vi "ElevEnc.vi"(11 "Reset?":bool) -> (3 "ElevEnc":dbl)   [LabVIEW 2017]
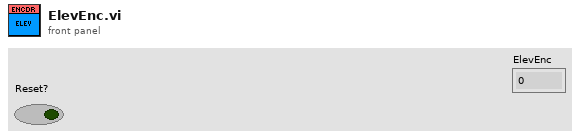
[diagram p1: front panel]
types:
  T1 = typedef "WPI_EncoderDevRef.ctl" = cluster{"DevStatus":errorcluster, "EncoderIndex":T2, "CounterIndex":T3, "DistancePerCount":dbl, "Decoding Type":T4}
  T2 = typedef "FPGA_EncoderIdx.ctl" = enum8{"Enc 0", "Enc 1", "Enc 2", "Enc 3", "Enc 4", "Enc 5", "Enc 6", "Enc 7", "Invalid"}
  T3 = typedef "FPGA_CounterCtrSystemIndex.ctl" = enum8{"Ctr 0", "Ctr 1", "Ctr 2", "Ctr 3", "Ctr 4", "Ctr 5", "Ctr 6", "Ctr 7", "Invalid"}
  T4 = typedef "WPI_EncoderType.ctl" = enum16{"1x", "2x", "4x"}
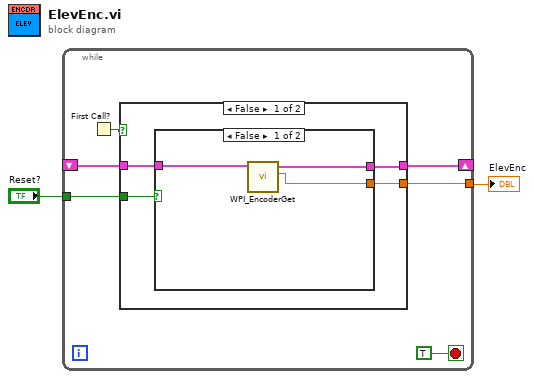
[diagram p0: block diagram]
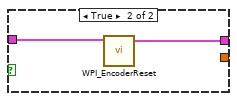
[diagram p2: hidden frame]
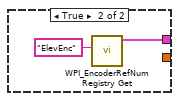
[diagram p3: hidden frame]
diagram:
  n1 = while {
    shift-right: [w6] -> _
    shift-left: _ -> [w5]
    tunnel: "Reset?" -> [w4]
    tunnel: [w3] -> w1
    stop <- TRUE stop-if-true
    n2 = First Call?() -> (First Call?: T/F=w8:bool)
    n3 = case shown="False" w8 {
      tunnel: [w10 w18] -> w6
      tunnel: w5 -> [w11 _]
      tunnel: w4 -> [w12 _]
      tunnel: [w9 _] -> w3
      frame False {
        n4 = case shown="False" w12 {
          tunnel: w11 -> [w15 w17]
          tunnel: [w14 w16] -> w10
          tunnel: [w13 _] -> w9
          frame False {
            n5 = call <vilib>:"WPI_EncoderGet.vi"("EncoderDevRef"=w15) -> ("Distance"=w13:dbl, "EncoderDevRef"=w14:T1)  [unwired: 5 in, 4 out]
          }
          frame True {
            n6 = call <vilib>:"WPI_EncoderReset.vi"("EncoderDevRef"=w17) -> ("EncoderDevRef"=w16:T1)  [unwired: 9 in, 1 out]
          }
        }
      }
      frame True {
        n7 = call <vilib>:"WPI_EncoderRefNum Registry Get.vi"("refnum name"="ElevEnc") -> ("EncoderDevRef"=w18:T1)  [unwired: 9 in, 1 out]
      }
    }
  }
  "ElevEnc" <- w1
